vi "基于延迟的串口通信组件.(Master)vi.vi"(0 "查询":string(combo)="CH0", 5 "error in":errorcluster) -> (14 "读取缓冲区":string, 19 "error out":errorcluster)   [LabVIEW 2013]
uses:
  <vilib>/Instr/_visa.llb/VISA Configure Serial Port (Instr).vi
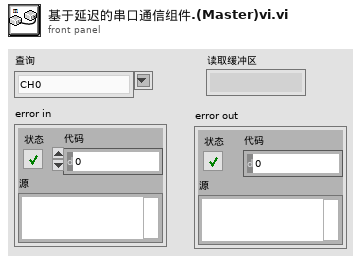
[diagram p1: front panel]
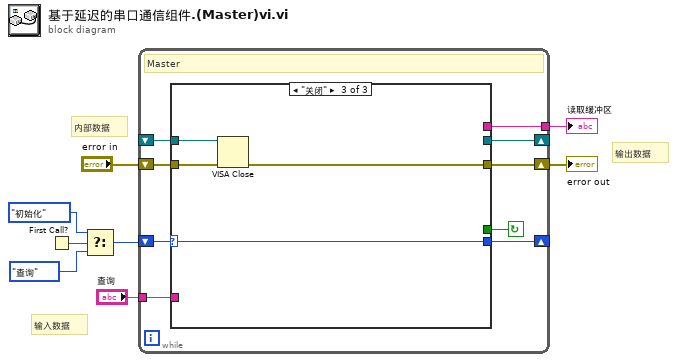
[diagram p0: block diagram]
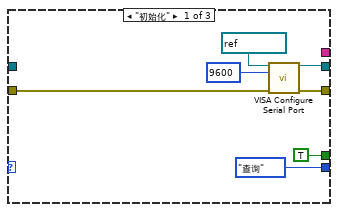
[diagram p2: hidden frame]
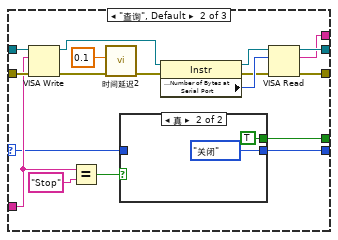
[diagram p3: hidden frame]
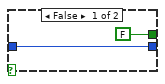
[diagram p4: hidden frame]
diagram:
  # "内部数据"
  # "输出数据"
  # "输入数据"
  n1 = First Call?() -> (First Call?: T/F=w5:bool)
  n2 = Select(t=enum16{"初始化", "空闲", "查询", "关闭"}."初始化" ("枚举"), s=w5, f=enum16{"初始化", "空闲", "查询", "关闭"}."查询" ("枚举")) -> (s? t:f=w4:enum16{"初始化", "空闲", "查询", "关闭"})
  n3 = while {
    shift-right: [w17] -> w1
    shift-left: "error in" -> [w15]
    shift-right: [w16] -> _
    shift-left: _ -> [w14]
    tunnel: "查询" -> [w13]
    tunnel: [w12] -> w7
    shift-right: [w9] -> _
    shift-left: w4 -> [w10]
    stop <- w11 continue-if-true
    # "Master"
    n4 = case shown="\"关闭\"" w10 {
      selector: w10 -> [_ w27 w47]
      tunnel: [w22 w33 _] -> w16
      tunnel: [w21 w32 w49] -> w17
      tunnel: w15 -> [w20 w34 w50]
      tunnel: w14 -> [_ w35 w48]
      tunnel: w13 -> [_ w30 _]
      tunnel: [_ w31 _] -> w12
      tunnel: [TRUE w25 _] -> w11
      tunnel: [enum16{"初始化", "空闲", "查询", "关闭"}."查询" ("枚举") w26 w47] -> w9
      frame "初始化" {
        n5 = call-poly "VISA Configure Serial Port"("VISA resource name"=refnum<visa-resource-name> "COM2", "baud rate (9600)"=u32 9600, "error in (no error)"=w20) -> ("VISA resource name out"=w22:refnum<visa-resource-name>, "error out"=w21:errorcluster)  [unwired: 11 in]
      }
      frame "查询", Default {
        n6 = VISA Write(VISA resource name=w35, write buffer=w30, error in (no error)=w34) -> (VISA resource name out=w39:refnum<visa-resource-name>, error out=w37:errorcluster)  [unwired: 1 out]
        n7 = Equal?(x=w30, y="Stop") -> (x = y?=w28:bool)
        n8 = call "时间延迟2"("error in (no error)"=w37, "Delay Time (s)"=0.1) -> ("error out"=w38:errorcluster)  [unwired: 9 in]
        n9 = case shown="真" w28 {
          tunnel: w27 -> [w44 _]
          tunnel: [w44 enum16{"初始化", "空闲", "查询", "关闭"}."关闭"] -> w26
          tunnel: [FALSE TRUE] -> w25
          frame False {
          }
          frame True {
          }
        }
        n10 = property class="Instr"(reference=w39, error in=w38) -> (reference out=w40:refnum<visa-resource-name>, error out=w41:errorcluster, "Serial Settings:Number of Bytes at Serial Port"=w42:u32)
        n11 = VISA Read(VISA resource name=w40, byte count=w42, error in (no error)=w41) -> (VISA resource name out=w33:refnum<visa-resource-name>, read buffer=w31:string, error out=w32:errorcluster)  [unwired: 1 out]
      }
      frame "关闭" {
        n12 = VISA Close(VISA resource name=w48, error in (no error)=w50) -> (error out=w49:errorcluster)
      }
    }
  }
  "读取缓冲区" <- w7
  "error out" <- w1
